vi "WebSocket Server Connection Handler.vi"(8 "error in (no error)":errorcluster, 11 "WebSocket in":refnum<class "WebSocket.lvclass">) -> (0 "error out":errorcluster)   [LabVIEW 2019]
uses:
  <vilib>/mediamongrels ltd/websockets/websockets/websocket/WebSocket.lvclass
panel:
  out "Received":cluster{"deltaT":u32, "buffer":string}[](array[cluster])
  in  "Filter SimDev":bool
  in  "Trace":bool
  out "Received Data":string
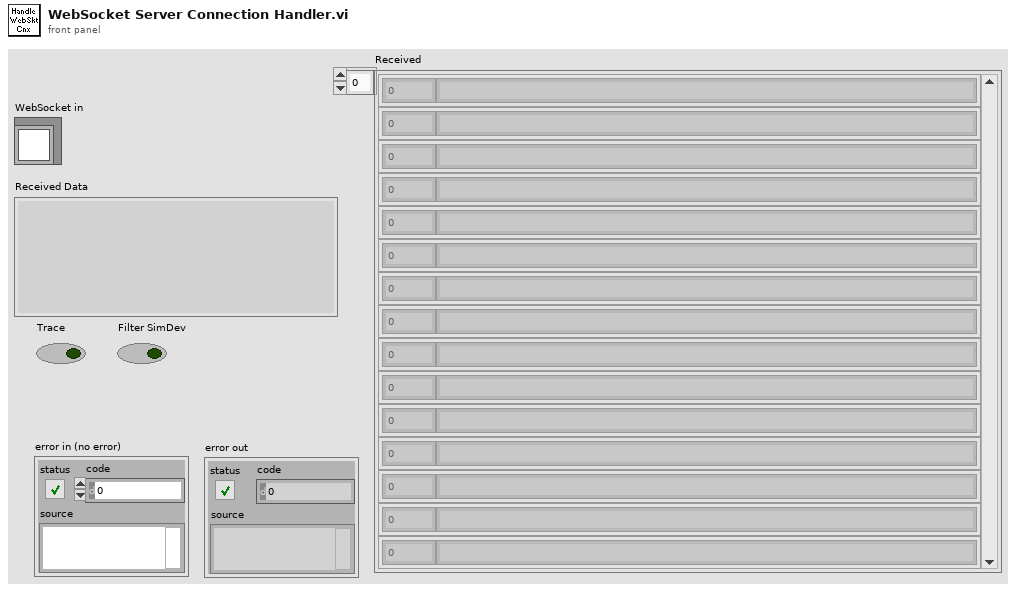
[diagram p1: front panel]
types:
  T1 = enum16{"add client", "remove client", "get clients", "clear"}
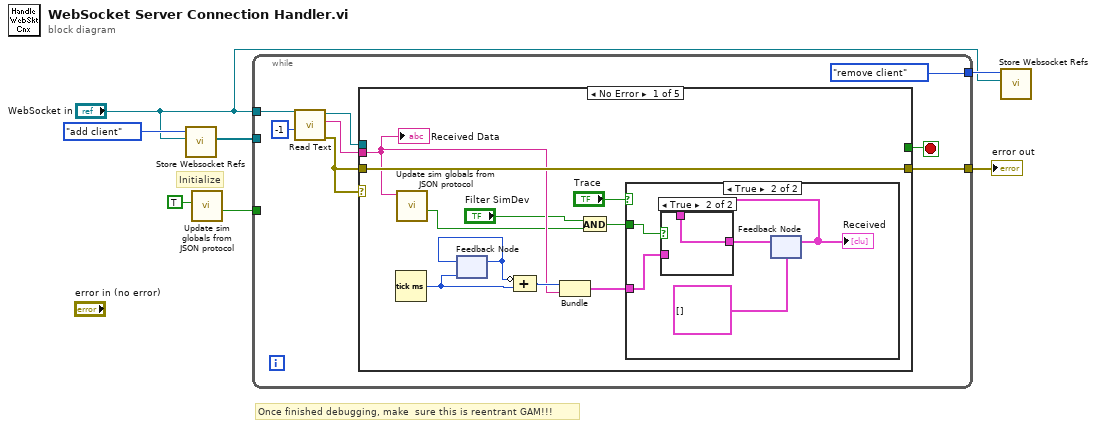
[diagram p0: block diagram]
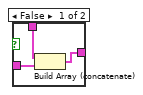
[diagram p3: hidden frame]
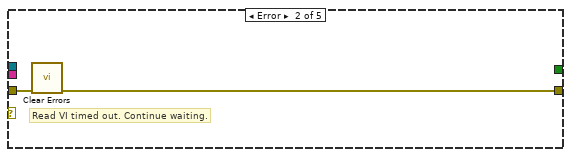
[diagram p4: hidden frame]
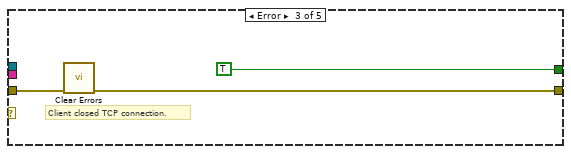
[diagram p5: hidden frame]
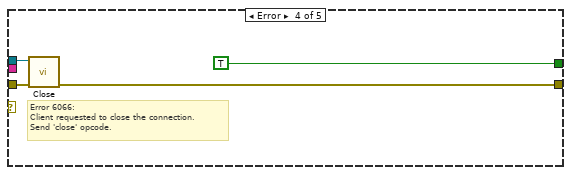
[diagram p6: hidden frame]
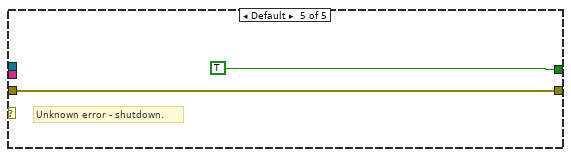
[diagram p7: hidden frame]
diagram:
  # "Initialize"
  # "Once finished debugging, make  sure this is reentrant GAM!!!"
  n1 = call "Store Websocket Refs.vi"("WebSocket in"="WebSocket in", "menu"=T1."add client") -> ("Clients"=w1:refnum<class "WebSocket.lvclass">[])  [unwired: 9 in]
  n2 = call "Update sim globals from JSON protocol.vi"("Initialize"=TRUE) -> ("SimDevice"=w4:bool)  [unwired: 10 in]
  n3 = while {
    tunnel: "WebSocket in" -> [w15]
    tunnel: [T1."remove client" ("menu")] -> w7
    tunnel: [w8] -> w6
    tunnel: w4 -> [_]
    tunnel: w1 -> [_]
    stop <- w10 stop-if-true
    n4 = call-dynamic "Read Text.vi"("timeout ms (5000)"=-1, "WebSocket in"=w15) -> ("error out"=w13:errorcluster, "Data"=w11:string, "WebSocket out"=w12:refnum<class "WebSocket.lvclass">)  [unwired: 7 in]
    n5 = case shown="No Error" w13 {
      tunnel: w11 -> [w21 _ _ _ _]
      tunnel: [_ _ TRUE TRUE TRUE] -> w10
      tunnel: w12 -> [_ _ _ w43 _]
      tunnel: w13 -> [w25 w36 w38 w41 w44]
      tunnel: [w25 w35 w37 w40 w44] -> w8
      frame No Error {
        n6 = Tick Count (ms)() -> (millisecond timer value=w23:u32)
        n7 = call "Update sim globals from JSON protocol.vi"("Data"=w21) -> ("SimDevice"=w17:bool)  [unwired: 10 in]
        n8 = feedback #1(w23) -> (w24:u32)
        n9 = feedback-in #1(w24) -> ()
        n10 = Compound Arithmetic op=ADD(invert w24, w23) -> (w22:u32)
        n11 = Bundle(w22, "Data"=w21) -> (w19:cluster{u32, "Data":string})  [unwired: 1 in]
        n12 = And(x="Filter SimDev", y=w17) -> (x .and. y?=w18:bool)
        n13 = case shown="True" "Trace" {
          tunnel: w19 -> [_ w29]
          tunnel: w18 -> [_ w30]
          frame False {
          }
          frame True {
            n14 = feedback #2(cluster{u32, "Data":string}[] []) -> (w26:cluster{u32, "Data":string}[])
            "Received" <- w26
            n15 = case shown="True" w30 {
              tunnel: w26 -> [w33 w34]
              tunnel: w29 -> [w32 _]
              tunnel: [w31 w34] -> w28
              frame False {
                n16 = Build Array (concatenate)(w33, w32) -> (w31:cluster{u32, "Data":string}[])
              }
              frame True {
              }
            }
            n17 = feedback-in #2(w28) -> ()
          }
        }
        "Received Data" <- w21
      }
      frame Error {
        # "Read VI timed out. Continue waiting."
        n18 = call <vilib>:"Clear Errors.vi"("error in (no error)"=w36) -> ("error out"=w35:errorcluster)  [unwired: 5 in, 1 out]
      }
      frame Error {
        # "Client closed TCP connection."
        n19 = call <vilib>:"Clear Errors.vi"("error in (no error)"=w38) -> ("error out"=w37:errorcluster)  [unwired: 5 in, 1 out]
      }
      frame Error {
        # "Error 6066:\nClient requested to close the connection.\nSend 'close' opcode."
        n20 = call-dynamic "Close.vi"("error in (no error)"=w41, "WebSocket in"=w43) -> ("error out"=w40:errorcluster)  [unwired: 9 in]
      }
      frame Default {
        # "Unknown error - shutdown."
      }
    }
  }
  "error out" <- w6
  n21 = call "Store Websocket Refs.vi"("WebSocket in"="WebSocket in", "menu"=w7) -> ()  [unwired: 9 in, 1 out]
